vi "New GoL.vi"(8 "error in":errorcluster, 11 "Grid":u8[][](array[numeric])) -> (0 "error out":errorcluster, 3 "GoL out":refnum<class "GoL.lvclass">)   [LabVIEW 2026, in "GoL.lvlib" / "GoL.lvclass"]
uses:
  GoL.lvclass
  GoL.lvclass/GoL.ctl
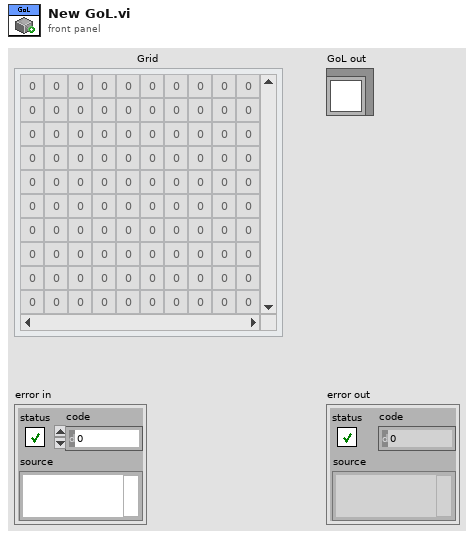
[diagram p1: front panel]
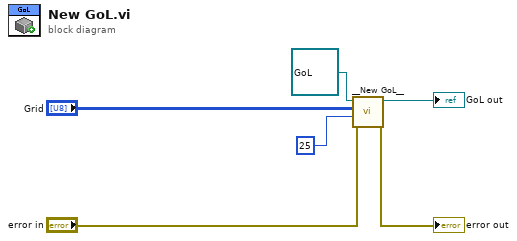
[diagram p0: block diagram]
diagram:
  n1 = call-dynamic "__New GoL__.vi"("error in"="error in", "Pixel Size"=i16 25, "Grid"="Grid", "GoL in"=refnum<class "GoL.lvclass"> refnum) -> ("error out"=→"error out":errorcluster, "GoL out"=→"GoL out":refnum<class "GoL.lvclass">)  [unwired: 6 in]
